vi "Set Setpoint.vi"(8 "error in (no error)":errorcluster, 10 "Setpoint Position":i32, 11 "IgusMotorDrive in":refnum<class "IgusMotorDrive.lvclass">) -> (0 "error out":errorcluster, 3 "IgusMotorDrive out":refnum<class "IgusMotorDrive.lvclass">)   [LabVIEW 2016, in "IgusMotorDrive.lvclass"]
uses:
  IgusMotorDrive.lvclass
  motor-drive/MotorDrive.lvclass
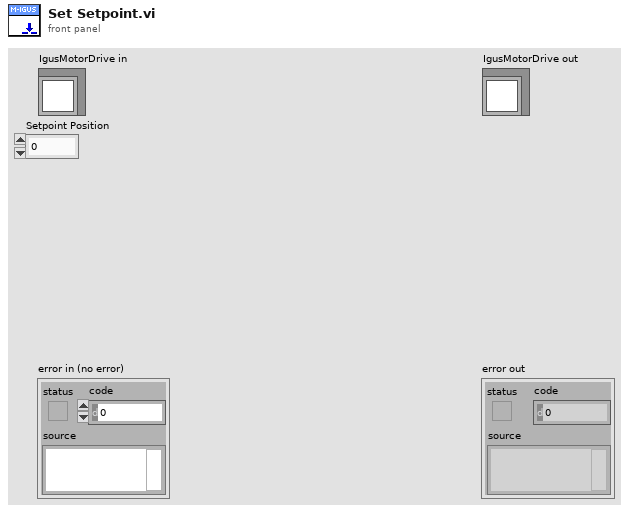
[diagram p1: front panel]
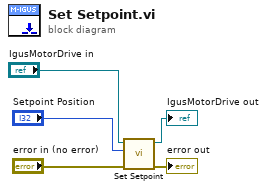
[diagram p0: block diagram]
diagram:
  n1 = call-parent "Set Setpoint.vi"("error in (no error)"="error in (no error)", "Setpoint Position"="Setpoint Position", "MotorDrive in"="IgusMotorDrive in") -> ("error out"=→"error out":errorcluster, "MotorDrive out"=→"IgusMotorDrive out":refnum<class "IgusMotorDrive.lvclass">)  [unwired: 7 in]
